vi "LvJDS2900_Sub_SetCommand.vi"(8 "error in (no error)":errorcluster caption="エラー入力（エラーなし）", 10 "Command":string, 11 "VISA rsrc":refnum<visa-resource-name>) -> (0 "error out":errorcluster caption="エラー出力", 3 "VISA rsrc out":refnum<visa-resource-name>)   [LabVIEW 2014]
panel:
  out "Response":string
  # ":w<nn>=<x>"
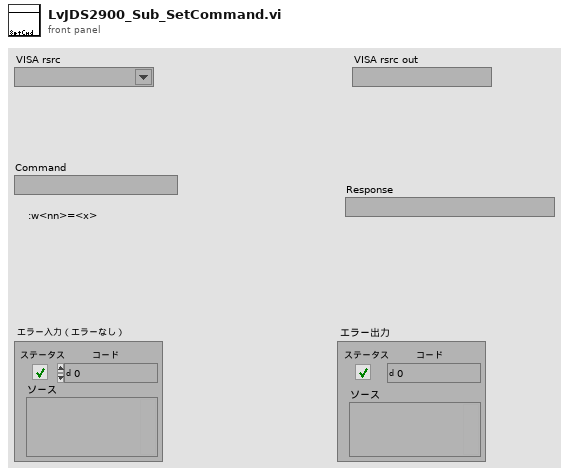
[diagram p1: front panel]
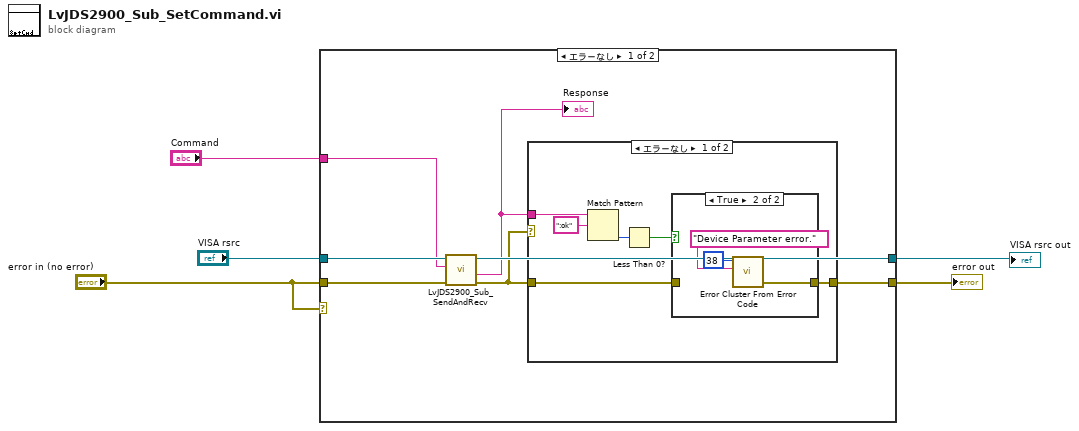
[diagram p0: block diagram]
diagram:
  n1 = case shown="エラーなし" "error in (no error)" {
    tunnel: "VISA rsrc" -> [w12 w24]
    tunnel: "Command" -> [w9 _]
    tunnel: [w7 w25] -> w3
    tunnel: "error in (no error)" -> [w10 w25]
    tunnel: [w11 w24] -> w2
    frame No Error {
      n2 = call "LvJDS2900_Sub_SendAndRecv.vi"("error in (no error)"=w10, "Command"=w9, "VISA rsrc"=w12) -> ("error out"=w8:errorcluster, "Response"=w6:string, "VISA rsrc out"=w11:refnum<visa-resource-name>)  [unwired: 6 in]
      "Response" <- w6
      n3 = case shown="エラーなし" w8 {
        tunnel: w6 -> [w18 _]
        tunnel: w8 -> [w14 w23]
        tunnel: [w13 w23] -> w7
        frame No Error {
          n4 = Match Pattern(string=w18, regular expression=":ok" ("正規表現")) -> (offset past match=w16:i32)  [unwired: 1 in, 3 out]
          n5 = Less Than 0?(x=w16) -> (x < 0?=w15:bool)
          n6 = case shown="TRUE" w15 {
            tunnel: w14 -> [w19 _]
            tunnel: [w19 w20] -> w13
            frame False {
            }
            frame True {
              n7 = call <vilib>:"Error Cluster From Error Code.vi"("error message (\"\")"="Device Parameter error." ("error message (\"\")"), "error code (0)"=38) -> ("error out"=w20:errorcluster)  [unwired: 7 in]
            }
          }
        }
        frame Error {
        }
      }
    }
    frame Error {
    }
  }
  "error out" <- w3
  "VISA rsrc out" <- w2
